vi "全局 1.vi"() -> ()   [LabVIEW 2020]
panel:
  out "逆开始":u32
  out "正结束":dbl
  out "正开始":u32
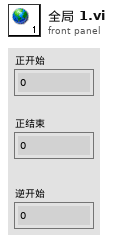
[diagram p1: front panel]
diagram:
